vi "Configure Voltage (Autorange).vi"(8 "error in (no error)":errorcluster, 10 "Autorange (On)":enum16{"Off", "On", "Once"}(ring)=enum."On", 11 "VISA resource name":refnum<visa-resource-name>) -> (0 "error out":errorcluster, 3 "VISA resource name out":refnum<visa-resource-name>)   [LabVIEW 2017, in "Keithley 3390.lvlib"]
doc: "Turns the function generator's auto ranging function on or off."
uses:
  Keithley 3390.lvlib
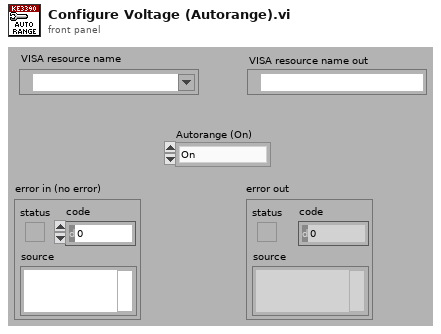
[diagram p1: front panel]
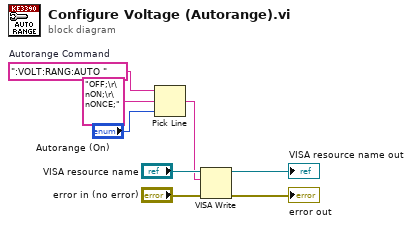
[diagram p0: block diagram]
diagram:
  w3 = ":VOLT:RANG:AUTO "  # Autorange Command
  n1 = Pick Line(string ("")=w3, multi-line string="OFF;\r\nON;\r\nONCE;" ("options"), line index="Autorange (On)") -> (output string=w5:string)
  n2 = VISA Write(VISA resource name="VISA resource name", write buffer=w5, error in (no error)="error in (no error)") -> (VISA resource name out=→"VISA resource name out":refnum<visa-resource-name>, error out=→"error out":errorcluster)  [unwired: 1 out]
